vi "Write Logged Data.vi"(8 "error in":errorcluster, 10 "Data":T1[](array[typedef]) {"type" format="%04x"; "activity" format="%04x"; "error" format="%04x"; "cwd1" format="%04x"; "cwd2" format="%04x"; "swd1" format="%04x"; "swd2" format="%04x"; "data" format="%04x"}, 11 "CSV Word Logger in":refnum<class "CSV Word Logger.lvclass">) -> (0 "error out":errorcluster, 3 "CSV Word Logger out":refnum<class "CSV Word Logger.lvclass">)   [LabVIEW 2020, in "Ballard MIL-STD-1553 Engine.lvlib" / "Implementation.lvlib" / "CSV Word Logger.lvclass"]
uses:
  CSV Word Logger.lvclass
  Word.ctl
  CSV Word Logger.lvclass/CSV Word Logger.ctl
  3e68417c-88ea-46f3-a078-ba49f2c6225d.vi
  Implementation.lvlib
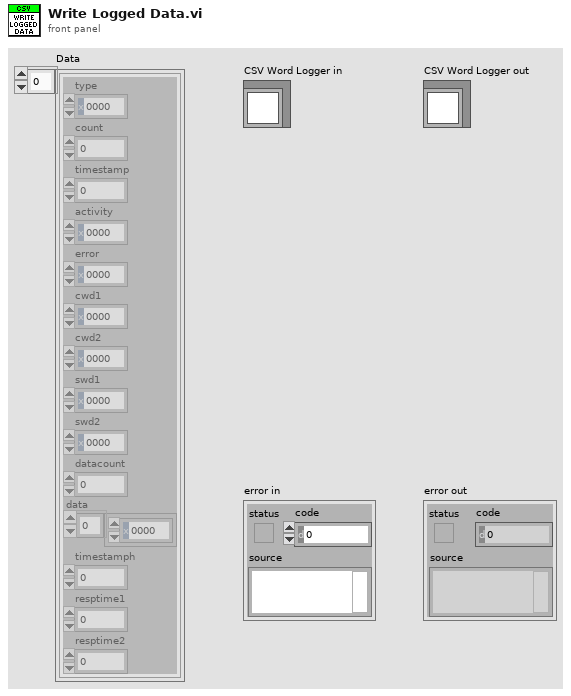
[diagram p1: front panel]
types:
  T1 = typedef "Ballard MIL-STD-1553 Engine.lvlib/Implementation.lvlib/Word.ctl" = cluster{"type":u16, "count":u16, "timestamp":u32, "activity":u16, "error":u16, "cwd1":u16, "cwd2":u16, "swd1":u16, "swd2":u16, "datacount":u16, "data":u16[], "timestamph":u32, "resptime1":u16, "resptime2":u16}
  T2 = typedef "Data Word Format.ctl" = string
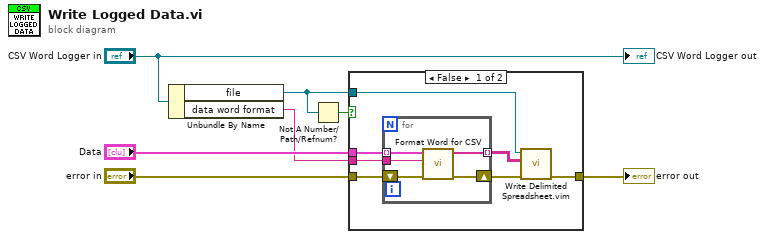
[diagram p0: block diagram]
diagram:
  n1 = Unbundle By Name("CSV Word Logger in") -> ("file"=w4:refnum<file>, "data word format"=w2:T2)
  n2 = Not A Number/Path/Refnum?(number/path/refnum=w4) -> (NaN/Path/Refnum?=w3:bool)
  n3 = case shown="False" w3 {
    tunnel: "Data" -> [w14 _]
    tunnel: w4 -> [w12 _]
    tunnel: [w11 w20] -> w5
    tunnel: w2 -> [w10 _]
    tunnel: "error in" -> [w9 w20]
    frame False {
      n4 = for {
        tunnel: w14 -> [w19] mode=indexing
        tunnel: [w18] -> w13 mode=indexing
        tunnel: w10 -> [w17]
        shift-right: [w15] -> w8
        shift-left: w9 -> [w16]
        n5 = call "Format Word for CSV.vi"("error in"=w16, "Data Word Format"=w17, "Word"=w19) -> ("error out"=w15:errorcluster, "String Array"=w18:string[])  [unwired: 7 in]
      }
      n6 = call "Write Delimited Spreadsheet.vim"("error in (no error)"=w8, "data"=w13, "file in"=w12) -> ("error out"=w11:errorcluster)  [unwired: 7 in, 1 out]
    }
    frame True {
    }
  }
  "error out" <- w5
  "CSV Word Logger out" <- "CSV Word Logger in"
